vi "local variable_kitchen timer.vi"() -> ()   [LabVIEW 2016]
panel:
  in  "Timer":i16(knob) scale=0.0..10.0
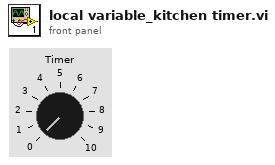
[diagram p1: front panel]
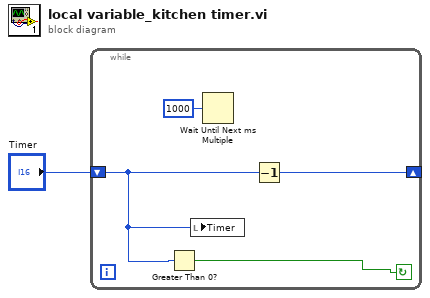
[diagram p0: block diagram]
diagram:
  n1 = while {
    shift-right: [w4] -> _
    shift-left: "Timer" -> [w3]
    stop <- w2 continue-if-true
    n2 = Greater Than 0?(x=w3) -> (x > 0?=w2:bool)
    n3 = local write "Timer"(w3) -> ()
    n4 = Wait Until Next ms Multiple(millisecond multiple=u32 1000) -> ()  [unwired: 1 out]
    n5 = Decrement(x=w3) -> (x-1=w4:i16)
  }
